vi "Measuring moving average.vi"() -> ()   [LabVIEW 2020]
uses:
  <vilib>/ptbypt/NI_PtbyPt.lvlib
panel:
  out "Waveform Chart":cluster{dbl, "number: 0 to 1":dbl, "mean":dbl}(graph)={0.47438739426612225, "number: 0 to 1"=0.7489711019122182, "mean"=0.47438739426612236}
  out "mean":dbl=0.43836561209050534 format="%0.2f"
  in  "stop":bool
  in  "Sample size to average over":i32=1000
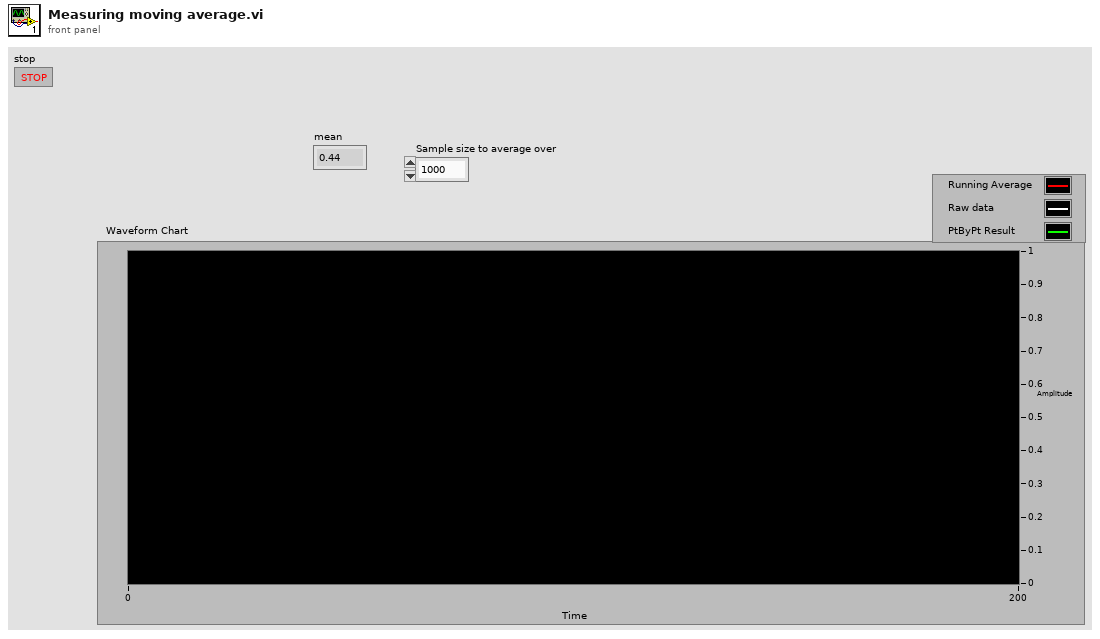
[diagram p1: front panel]
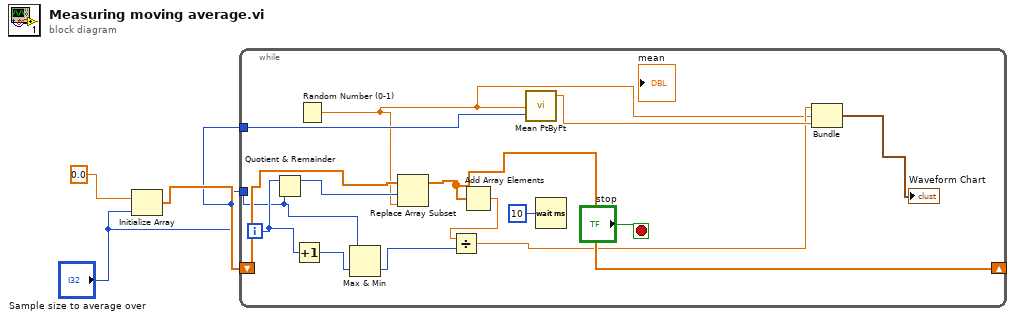
[diagram p0: block diagram]
diagram:
  n1 = Initialize Array(0.0 ("element"), "Sample size to average over") -> (w3:dbl[])
  n2 = while {
    tunnel: "Sample size to average over" -> [w9]
    shift-right: [w14] -> _
    shift-left: w3 -> [w16]
    tunnel: "Sample size to average over" -> [w11]
    i -> [w12]
    stop <- "stop" stop-if-true
    n3 = Quotient & Remainder(x=w12, y=w9) -> (x-y*floor(x/y)=w15:i32)  [unwired: 1 out]
    n4 = Increment(x=w12) -> (x+1=w10:i32)
    n5 = Random Number (0-1)() -> (number: 0 to 1=w5:dbl)
    n6 = Max & Min(x=w9, y=w10) -> (min(x,y)=w8:i32)  [unwired: 1 out]
    n7 = Replace Array Subset(array=w16, new element=w5, index=w15) -> (w14:dbl[])
    n8 = Add Array Elements(numeric array=w14) -> (sum=w13:dbl)
    n9 = Divide(x=w13, y=w8) -> (x/y=w6:dbl)
    n10 = call <vilib>:"Mean PtByPt.vi"("x"=w5, "sample length"=w11) -> ("mean"=w7:dbl)  [unwired: 2 in, 1 out]
    n11 = Wait (ms)(milliseconds to wait=u32 10) -> ()  [unwired: 1 out]
    n12 = Bundle(w6, "number: 0 to 1"=w5, "mean"=w7) -> (→"Waveform Chart":cluster{dbl, "number: 0 to 1":dbl, "mean":dbl})  [unwired: 1 in]
  }
